vi "Get - Time Data OBJ State.vi"(0 "reference in":refnum<class "TEXT.lvclass">, 5 "error in (no error)":errorcluster) -> (13 "New Time Data Obj?":bool, 14 "reference out":refnum<class "TEXT.lvclass">, 19 "error out":errorcluster)   [LabVIEW 2022 SP3, in "TEXT.lvclass"]
uses:
  TEXT.lvclass
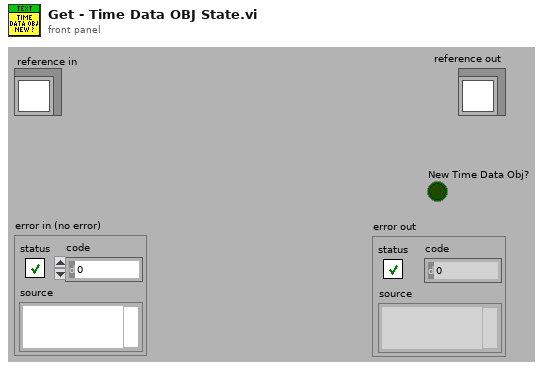
[diagram p1: front panel]
types:
  T1 = typedef "TEXT.lvclass/ObjectAttributes.ctl" = cluster{"Time Data":refnum<class "GSwFormDSP.lvclass">, "New Time Data Obj?":bool}
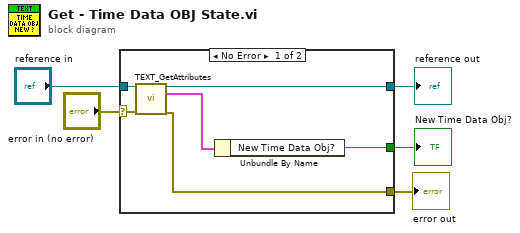
[diagram p0: block diagram]
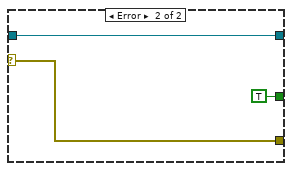
[diagram p2: hidden frame]
diagram:
  n1 = case shown="No Error" "error in (no error)" {
    selector: "error in (no error)" -> [w11 w14]
    tunnel: [w10 w14] -> w4
    tunnel: [w9 w13] -> w2
    tunnel: "reference in" -> [w7 w13]
    tunnel: [w6 TRUE ("New Time Data Obj?")] -> w1
    frame No Error {
      n2 = call "TEXT_GetAttributes.vi"("reference in"=w7, "error in (no error)"=w11) -> ("reference out"=w9:refnum<class "TEXT.lvclass">, "attributes"=w8:T1, "error out"=w10:errorcluster)  [unwired: 14 in, 1 out]
      n3 = Unbundle By Name(w8) -> ("New Time Data Obj?"=w6:bool)
    }
    frame Error {
    }
  }
  "error out" <- w4
  "reference out" <- w2
  "New Time Data Obj?" <- w1
